vi "Core Housekeep.vi"(8 "error in (no error)":errorcluster, 11 "CIFCorePlugin in":refnum<class "CIFCorePlugin.lvclass">) -> (0 "error out":errorcluster, 3 "CIFCorePlugin out":refnum<class "CIFCorePlugin.lvclass">)   [LabVIEW 2021, in "CIFCorePlugin.lvclass"]
uses:
  CIFCorePlugin.lvclass
  Typedef/Energized States.ctl
  CIFCorePlugin.lvclass/CIFCorePlugin.ctl
  CIFUtilities/CIFOutOfBand/CIFOutOfBand.lvclass/CIFOutOfBand.ctl
  Common/Utilities/Update Cycle Time.vi
  Common/Utilities/Update Delta Time.vi
  Accessors/Timestamps/Write Housekeeping TS.vi
  Accessors/Get Time.vi
  Accessors/Timestamps/Read Execute TS.vi
  Accessors/Timestamps/Read Housekeeping TS.vi
  Accessors/Timestamps/Read Sleep TS.vi
  Accessors/Timestamps/Read Target Wake TS.vi
  OOB/OOB_Rx/Receive/Check for OOB Commands.vi
  OOB/OOB_Rx/Receive/Read FTE.vi
  SubVIs/Refresh Stats.vi
  OOB/OOB_Tx/Send/Update Status Command.vi
  OOB/OOB_Tx/Send/Update Override Command.vi
  CIFUtilities/CIFClocks/SubVIs/Add Error.vi
  CIFUtilities/CIFClocks/Core/Get Time.vi
  CIFUtilities/CIFOutOfBand/Read OOB DVR.vi
  OOB/OOB_Rx/Private/Command Settings.vi
  OOB/OOB_Rx/Private/Read Payload.vi
  CIFUtilities/CIFOutOfBand/Write OOB DVR.vi
  CIFUtilities/CIFOutOfBand/Utilities/Command to Bitwise Command.vi
  CIFUtilities/CIFOutOfBand/Accessors/Read Local OOB Data.vi
  CIFUtilities/CIFOutOfBand/Accessors/Write Local OOB Data.vi
  Common/Utilities/Append Error Location.vi
  CIFUtilities/CIFClocks/Time Conversion/LabVIEW Time to UTC Time.vi
  OOB/OOB_Tx/CIFCoreOOB_Tx.lvclass
  D:/dev/CIF-LVCore/src/CIFUtilities/CIFOutOfBand/CIFOutOfBand.lvclass
  OOB/OOB_Rx/CIFCoreOOB_Rx.lvclass
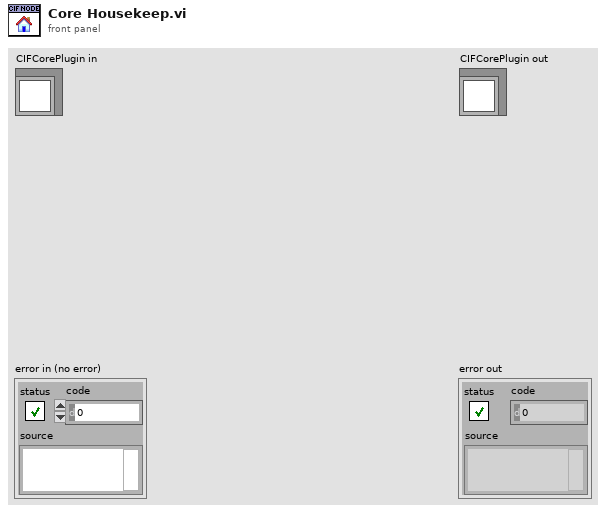
[diagram p1: front panel]
types:
  T1 = typedef "CIFCorePlugin.lvclass/Energized States.ctl" = enum16{"Listen", "Prepare", "Execute", "Housekeep", "Cleanup", "Destroy"}
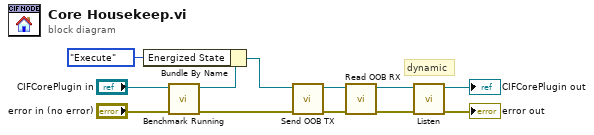
[diagram p0: block diagram]
diagram:
  # "dynamic"
  n1 = call "Benchmark Running.vi"("error in (no error)"="error in (no error)", "CIFCorePlugin in"="CIFCorePlugin in") -> ("error out"=w8:errorcluster, "CIFCorePlugin out"=w10:refnum<class "CIFCorePlugin.lvclass">)  [unwired: 8 in]
  n2 = Bundle By Name(cluster=w10, "Energized State"=Energized_States."Execute") -> (w12:refnum<class "CIFCorePlugin.lvclass">)
  n3 = call "Send OOB TX.vi"("error in (no error)"=w8, "CIFCorePlugin in"=w12) -> ("error out"=w6:errorcluster, "CIFCorePlugin out"=w7:refnum<class "CIFCorePlugin.lvclass">)  [unwired: 8 in]
  n4 = call "Read OOB RX.vi"("error in (no error)"=w6, "CIFCorePlugin in"=w7) -> ("error out"=w4:errorcluster, "CIFCorePlugin out"=w5:refnum<class "CIFCorePlugin.lvclass">)  [unwired: 8 in]
  n5 = call-dynamic "Listen.vi"("error in (no error)"=w4, "CIFTemplateNode in"=w5) -> ("error out"=→"error out":errorcluster, "CIFTemplateNode out"=→"CIFCorePlugin out":refnum<class "CIFCorePlugin.lvclass">)  [unwired: 8 in]
